vi "Trigger Timestamp.vi"(8 "error in (no error)":errorcluster, 11 "TrialBasedExperiment in":refnum<class "TrialBasedExperiment.lvclass">) -> (0 "error out":errorcluster, 3 "TrialBasedExperiment out":refnum<class "TrialBasedExperiment.lvclass">)   [LabVIEW 2014, in "AcquisitionCoreObjects.lvlib" / "TrialBasedExperiment.lvclass"]
uses:
  TrialBasedExperiment.lvclass
  <vilib>/DAQmx/create/channels.llb/DAQmx Create Channel (DO-Digital Output).vi
  <vilib>/DAQmx/write.llb/DAQmx Write (Digital Bool 1Line 1Point).vi
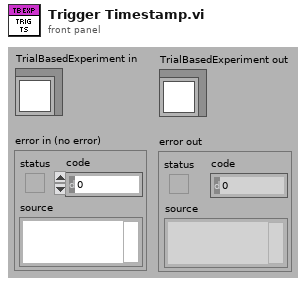
[diagram p1: front panel]
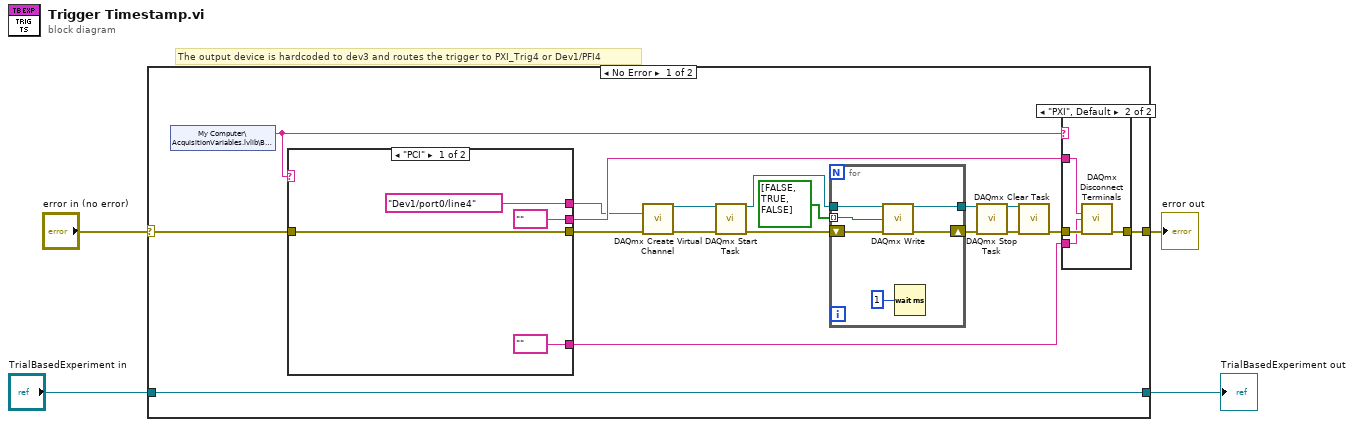
[diagram p0: block diagram]
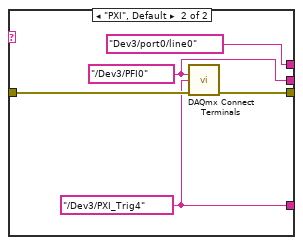
[diagram p3: hidden frame]
diagram:
  # "The output device is hardcoded to dev3 and routes the trigger to PXI_Trig4 or Dev1/PFI4"
  n1 = case shown="No Error" "error in (no error)" {
    selector: "error in (no error)" -> [w8 w44]
    tunnel: [w13 w44] -> w3
    tunnel: [w22 w43] -> w1
    tunnel: "TrialBasedExperiment in" -> [w22 w43]
    frame No Error {
      n2 = shared-variable "My Computer\\AcquisitionVariables.lvlib\\Bus System"() -> (w9:string)  [unwired: 1 in, 1 out]
      n3 = case shown="\"PCI\"" w9 {
        tunnel: [tag "" ("destination terminal") w34] -> w10
        tunnel: w8 -> [w30 w36]
        tunnel: [w30 w35] -> w7
        tunnel: [tag "" ("source terminal") w33] -> w6
        tunnel: [tag "Dev1/port0/line4" ("lines") tag "Dev3/port0/line0" ("lines")] -> w5
        frame "PCI" {
        }
        frame "PXI", Default {
          w33 = tag "/Dev3/PFI0" ("source terminal")
          w34 = tag "/Dev3/PXI_Trig4" ("destination terminal")
          n4 = call <vilib>:"DAQmx Connect Terminals.vi"("source terminal"=w33, "destination terminal"=w34, "error in"=w36) -> ("error out"=w35:errorcluster)  [unwired: 12 in]
        }
      }
      n5 = call-poly <vilib>:"DAQmx Create Virtual Channel.vi"("lines"=w5, "error in"=w7) -> ("task out"=w11:refnum<k21>, "error out"=w12:errorcluster)  [unwired: 12 in]
      n6 = call <vilib>:"DAQmx Start Task.vi"("task/channels in"=w11, "error in"=w12) -> ("task out"=w18:refnum<k21>, "error out"=w16:errorcluster)  [unwired: 12 out]
      n7 = for {
        tunnel: bool[] [FALSE, TRUE, FALSE] -> [w42] mode=indexing
        tunnel: w18 -> [w41]
        tunnel: [w40] -> w17
        shift-right: [w37] -> w15
        shift-left: w16 -> [w38]
        n8 = call-poly <vilib>:"DAQmx Write.vi"("task/channels in"=w41, "data"=w42, "error in"=w38) -> ("task out"=w40:refnum<k21>, "error out"=w37:errorcluster)  [unwired: 1 in, 10 out]
        n9 = Wait (ms)(milliseconds to wait=u32 1) -> ()  [unwired: 1 out]
      }
      n10 = call <vilib>:"DAQmx Stop Task.vi"("task/channels in"=w17, "error in"=w15) -> ("task out"=w21:refnum<k21>, "error out"=w20:errorcluster)  [unwired: 12 out]
      n11 = call <vilib>:"DAQmx Clear Task.vi"("task in"=w21, "error in"=w20) -> ("error out"=w14:errorcluster)  [unwired: 13 out]
      n12 = case shown="\"PXI\", Default" w9 {
        tunnel: w6 -> [_ w27]
        tunnel: w14 -> [w23 w26]
        tunnel: [w23 w25] -> w13
        tunnel: w10 -> [_ w24]
        frame "PCI" {
        }
        frame "PXI", Default {
          n13 = call <vilib>:"DAQmx Disconnect Terminals.vi"("source terminal"=w27, "destination terminal"=w24, "error in"=w26) -> ("error out"=w25:errorcluster)  [unwired: 12 in]
        }
      }
    }
    frame Error {
    }
  }
  "error out" <- w3
  "TrialBasedExperiment out" <- w1
